vi "时间-温度曲线(子VI).vi"   [LabVIEW 2016, in "斯坦道CODMn.lvlib"]
uses:
  <vilib>/ptbypt/NI_PtbyPt.lvlib
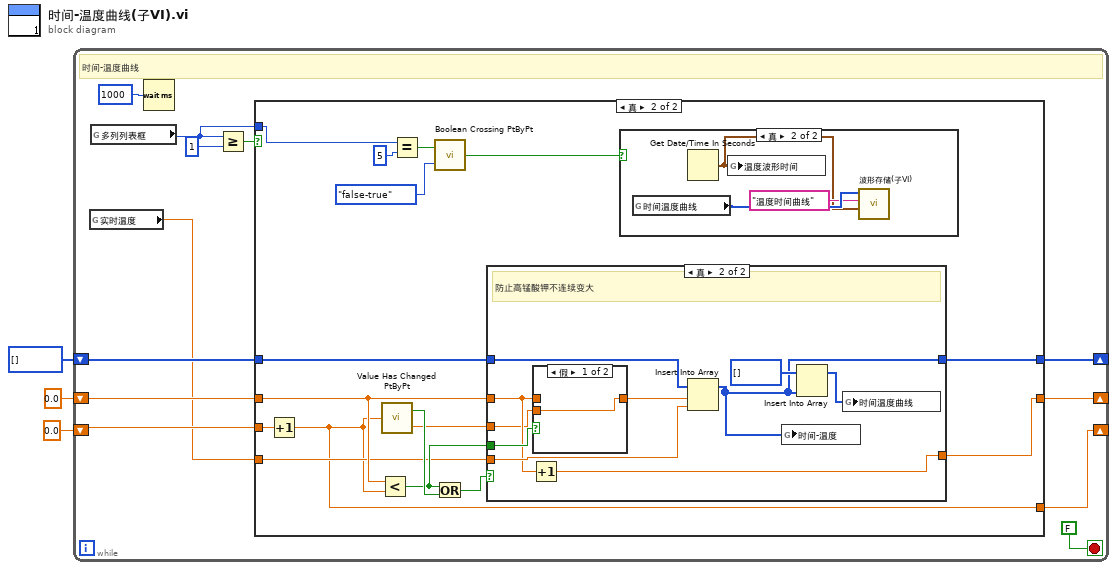
[diagram p0: block diagram]
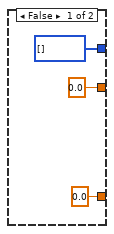
[diagram p2: hidden frame]
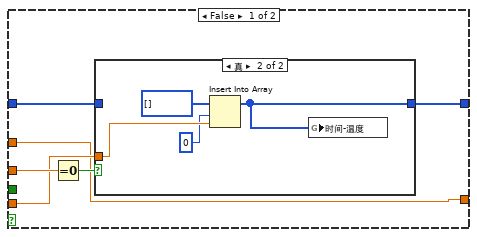
[diagram p4: hidden frame]
diagram:
  n1 = while {
    shift-right: [w12] -> _
    shift-left: u16[] [] ("ORP滴定曲线") -> [w13]
    shift-right: [w8] -> _
    shift-left: 0.0 -> [w9]
    shift-right: [w4] -> _
    shift-left: 0.0 -> [w6]
    stop <- FALSE stop-if-true
    # "时间-温度曲线"
    n2 = global read "COD内部交互全局.vi" "实时温度"() -> (w5:dbl)
    n3 = global read "运行时序全局变量.vi" "多列列表框"() -> (w7:i32)
    n4 = Wait (ms)(milliseconds to wait=u32 1000 ("等待时间（毫秒）")) -> ()  [unwired: 1 out]
    n5 = Greater Or Equal?(x=w7, y=1) -> (x >= y?=w10:bool)
    n6 = case shown="真" w10 {
      tunnel: w13 -> [_ w34]
      tunnel: [u16[] [] ("ORP滴定曲线") w33] -> w12
      tunnel: w9 -> [_ w25]
      tunnel: [0.0 w24] -> w8
      tunnel: w7 -> [_ w22]
      tunnel: w6 -> [_ w21]
      tunnel: w5 -> [_ w20]
      tunnel: [0.0 w19] -> w4
      frame False {
      }
      frame True {
        n7 = Increment(x=w21) -> (x+1=w19:dbl)
        n8 = Less?(x=w25, y=w19) -> (x < y?=w23:bool)
        n9 = call <vilib>:"Value Has Changed PtByPt.vi"("input data point"=w19) -> ("has changed"=w32:bool, "output data point"=w31:dbl)  [unwired: 1 in]
        n10 = Equal?(x=w22, y=5) -> (x = y?=w29:bool)
        n11 = call <vilib>:"Boolean Crossing PtByPt.vi"("direction"=enum16{"either", "false-true", "true-false"}."false-true", "input"=w29) -> ("crossing"=w27:bool)  [unwired: 1 in]
        n12 = Or(x=w23, y=w32) -> (x .or. y?=w26:bool)
        n13 = case shown="真" w26 {
          tunnel: w34 -> [w42 w57]
          tunnel: [w41 w49] -> w33
          tunnel: w31 -> [w43 w51]
          tunnel: w20 -> [w39 w56]
          tunnel: w25 -> [w38 w53]
          tunnel: [w38 w55] -> w24
          tunnel: w23 -> [_ w54]
          frame False {
            n14 = Equal To 0?(x=w43) -> (x = 0?=w40:bool)
            n15 = case shown="真" w40 {
              tunnel: [w44 w45] -> w41
              tunnel: w42 -> [w44 _]
              tunnel: w39 -> [_ w47]
              frame False {
              }
              frame True {
                n16 = Insert Into Array(array=u16[] [] ("ORP滴定曲线"), index=0 ("索引"), new element=w47) -> (w45:u16[])
                n17 = global write "COD内部交互全局.vi" "时间-温度"(w45) -> ()
              }
            }
          }
          frame True {
            # "防止高锰酸钾不连续变大"
            n18 = Increment(x=w53) -> (x+1=w55:dbl)
            n19 = case shown="假" w54 {
              tunnel: w53 -> [_ w60]
              tunnel: [w59 w60] -> w52
              tunnel: w51 -> [w59 _]
              frame False {
              }
              frame True {
              }
            }
            n20 = Insert Into Array(array=w57, index=w52, new element=w56) -> (w49:u16[])
            n21 = global write "COD内部交互全局.vi" "时间-温度"(w49) -> ()
            n22 = Insert Into Array(array=u16[] [] ("ORP滴定曲线"), new element=w49) -> (w50:u16[])  [unwired: 1 in]
            n23 = global write "COD内部交互全局.vi" "时间温度曲线"(w50) -> ()
          }
        }
        n24 = case shown="真" w27 {
          frame False {
          }
          frame True {
            n25 = global read "COD内部交互全局.vi" "时间温度曲线"() -> (w37:u16[])
            n26 = Get Date/Time In Seconds() -> (seconds since 1Jan1904=w35:timestamp)
            n27 = global write "COD内部交互全局.vi" "温度波形时间"(w35) -> ()
            n28 = call "波形存储(子VI).vi"("波形时间"=w35, "condition"="温度时间曲线", "ORP滴定曲线"=w37) -> ()  [unwired: 9 in]
          }
        }
      }
    }
  }
